vi "RSZVB Get Differential Mode Impedance.vi"(8 "error in (no error)":errorcluster {"code" format="%.0x"}, 9 "Logical Port (1)":i32=1, 10 "Channel (1)":i32=1, 11 "VISA session":refnum<visa-resource-name>) -> (0 "error out":errorcluster {"code" format="%.0x"}, 2 "Impedance":dbl format="%^.3e", 3 "dup VISA session":refnum<visa-resource-name>)   [LabVIEW 2011]
doc: "This VI queries the differential mode impedance for selected balanced port.\n\nRemote-control command(s):\nCALCulate<Ch>:FSIMulator:BALun:DZConversion:BPORt<logical_port>:ZDIFferent[:R]?"
uses:
  _utility/RSZVB Global Data.vi
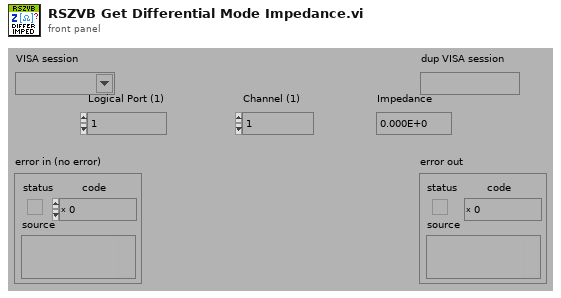
[diagram p1: front panel]
types:
  T1 = cluster{"Error Checking (T: On)":bool, "Installed Options":string[], "Data Valid?":bool, "Ports":i32, "Model":string[], "Option Checking (T: On)":bool}[]
  T2 = cluster{"Error Checking (T: On)":bool, "Installed Options":string[], "Data Valid?":bool, "Ports":i32, "Model":string[], "Option Checking (T: On)":bool}
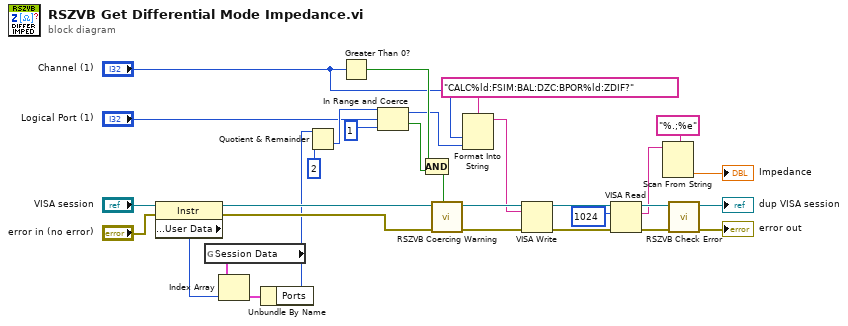
[diagram p0: block diagram]
diagram:
  n1 = property class="Instr"(reference="VISA session", error in="error in (no error)") -> (reference out=w19:refnum<visa-resource-name>, error out=w20:errorcluster, "General Settings:User Data"=w7:u32)
  n2 = global read "RSZVB Global Data.vi" "Session Data"() -> (w21:T1)
  n3 = Index Array(array=w21, index=w7) -> (element=w8:T2)
  n4 = Unbundle By Name(w8) -> ("Ports"=w13:i32)
  n5 = Quotient & Remainder(x=w13, y=2) -> (floor(x/y)=w15:i32)  [unwired: 1 out]
  n6 = Greater Than 0?(x="Channel (1)") -> (x > 0?=w22:bool)
  n7 = In Range and Coerce(upper limit=w15, x="Logical Port (1)", lower limit=1) -> (coerced(x)=w14:i32, In Range?=w17:bool)
  n8 = Compound Arithmetic op=AND(w22, w17) -> (w23:bool)
  n9 = call "RSZVB Coercing Warning.vi"("In Range?"=w23, "error in (no error)"=w20, "VISA session"=w19) -> ("error out"=w9:errorcluster, "dup VISA session"=w10:refnum<visa-resource-name>)  [unwired: 7 in]
  n10 = Format Into String(format string="CALC%ld:FSIM:BAL:DZC:BPOR%ld:ZDIF?", "Channel (1)", w14) -> (resulting string=w1:string)  [unwired: 2 in, 1 out]
  n11 = VISA Write(VISA resource name=w10, write buffer=w1, error in (no error)=w9) -> (VISA resource name out=w11:refnum<visa-resource-name>, error out=w12:errorcluster)  [unwired: 1 out]
  n12 = VISA Read(VISA resource name=w11, byte count=u32 1024 ("byte count (0)"), error in (no error)=w12) -> (VISA resource name out=w30:refnum<visa-resource-name>, read buffer=w27:string, error out=w29:errorcluster)  [unwired: 1 out]
  n13 = Scan From String(format string="%.;%e", input string=w27) -> (output 1=→"Impedance":dbl)  [unwired: 3 in, 3 out]
  n14 = call "RSZVB Check Error.vi"("error in (no error)"=w29, "VISA session"=w30) -> ("error out"=→"error out":errorcluster, "dup VISA session"=→"dup VISA session":refnum<visa-resource-name>)  [unwired: 8 in]
